vi "Release Semaphore Reference.vi"(8 "error in (no error)":errorcluster, 9 "force destroy? (F)":bool, 11 "semaphore":T1) -> (0 "error out":errorcluster, 3 "semaphore name":string)   [LabVIEW 2020]
doc: "Releases a reference to a semaphore."
uses:
  Semaphore Refnum Core.ctl
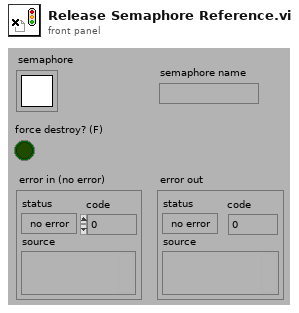
[diagram p1: front panel]
types:
  T1 = typedef "Semaphore RefNum" = refnum<k1>
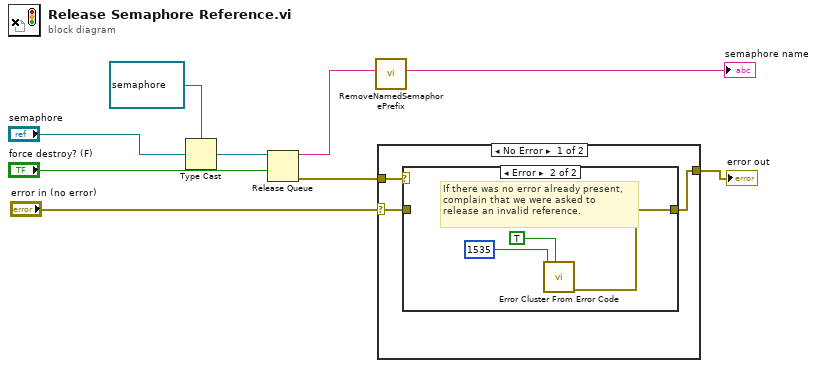
[diagram p0: block diagram]
diagram:
  w7 = refnum<queue> refnum items=["Semaphore Core"] ("queue out")
  n1 = Type Cast(type=w7, x="semaphore") -> (*(type *) &x=w6:refnum<queue>)
  n2 = Release Queue(queue=w6, force destroy? (F)="force destroy? (F)") -> (queue name=w1:string, error out=w5:errorcluster)  [unwired: 1 in, 1 out]
  n3 = call "RemoveNamedSemaphorePrefix.vi"("Name In"=w1) -> ("Name Out"=→"semaphore name":string)  [unwired: 10 out]
  n4 = case shown="No Error" "error in (no error)" {
    selector: "error in (no error)" -> [w10 w17]
    tunnel: [w12 w17] -> w4
    tunnel: w5 -> [w11 _]
    frame No Error {
      n5 = case shown="Error" w11 {
        tunnel: [w13 w14] -> w12
        tunnel: w10 -> [w13 _]
        frame No Error {
        }
        frame Error {
          # "If there was no error already present, \ncomplain that we were asked to \nrelease an invalid reference."
          n6 = call "Error Cluster From Error Code.vi"("show call chain? (False)"=TRUE, "error code (0)"=1535) -> ("error out"=w14:errorcluster)  [unwired: 1 in, 6 out]
        }
      }
    }
    frame Error {
      # "If there was an error present already, \ndon't overwrite it with one of our own."
    }
  }
  "error out" <- w4
